vi "Laplace.vi"() -> ()   [LabVIEW 2021]
uses:
  <vilib>/Math Plots/3D Math Plots/3D Contour/3D Contour XCtrl/3D Contour.xctl
  <vilib>/Math Plots/3D Math Plots/3D Contour/3D Contour Datatype/Public/Plot Helper (Matrix).vi
  <vilib>/Math Plots/3D Math Plots/3D Contour/3D Contour Datatype/3D Contour Datatype.lvclass
panel:
  out "abs(x) 2":dbl[][](array[numeric])
  out "abs(x)":dbl
  out "Boolean":bool
  in  "Error":dbl
  out "3D Contour":refnum<class "3D Plot Datatype.lvclass">[](xcontrol)
  in  "dimension size":i32
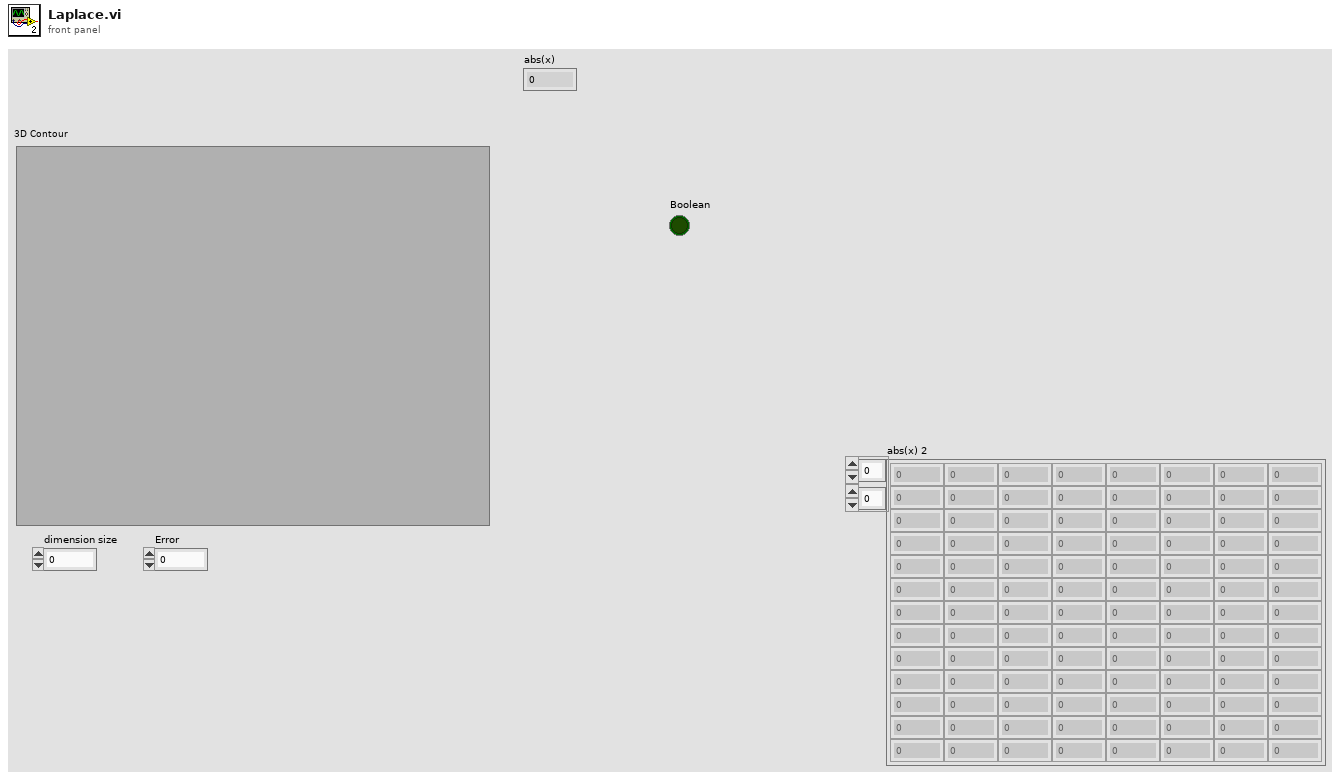
[diagram p1: front panel]
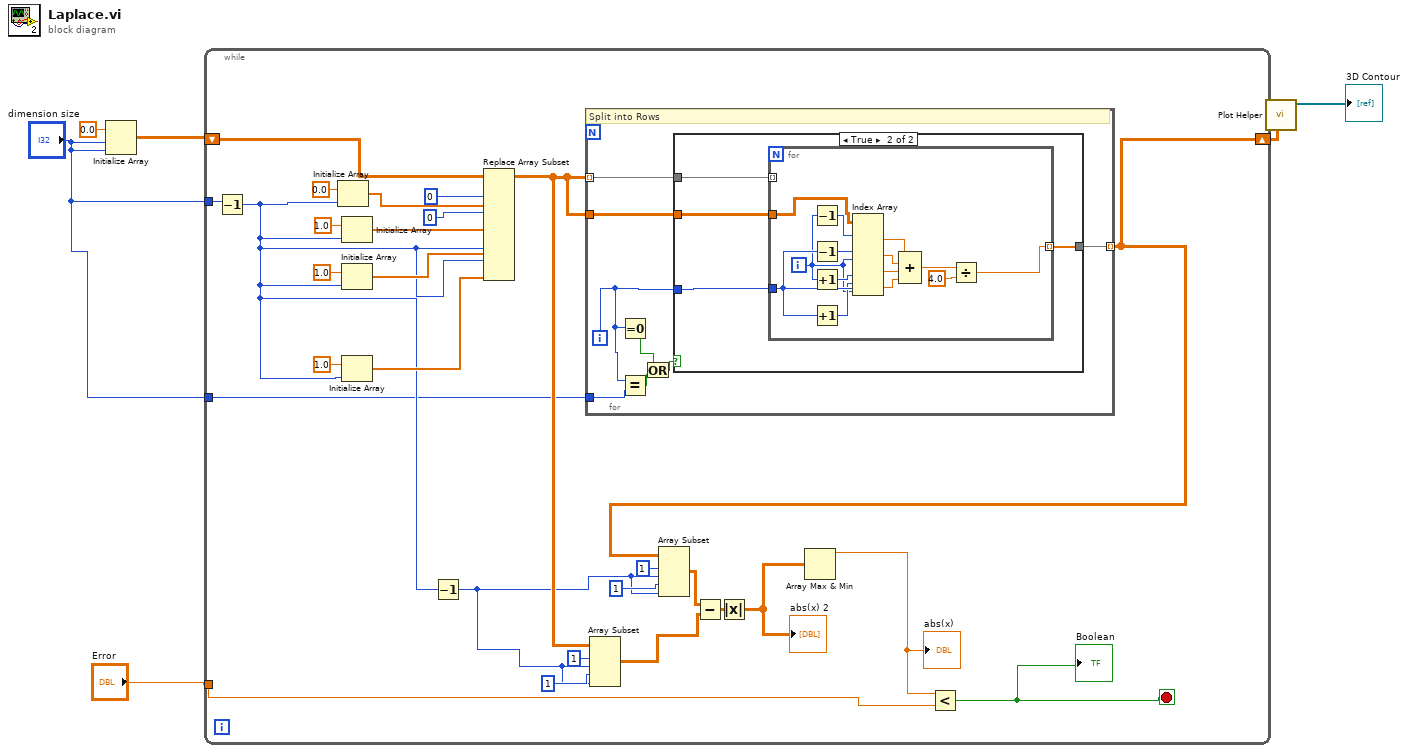
[diagram p0: block diagram]
diagram:
  n1 = Initialize Array(0.0 ("element"), "dimension size", "dimension size") -> (w5:dbl[][])
  n2 = while {
    tunnel: "dimension size" -> [w28]
    shift-right: [w12] -> w3
    shift-left: w5 -> [w29]
    tunnel: "Error" -> [w21]
    tunnel: "dimension size" -> [w7]
    stop <- w20 stop-if-true
    n3 = Decrement(x=w28) -> (x-1=w9:i32)
    n4 = Initialize Array(0.0 ("element"), w9) -> (w30:dbl[])
    n5 = Initialize Array(1.0 ("element"), w9) -> (w27:dbl[])
    n6 = Initialize Array(1.0 ("element"), w9) -> (w26:dbl[])
    n7 = Initialize Array(1.0 ("element"), w9) -> (w25:dbl[])
    n8 = Decrement(x=w9) -> (x-1=w8:i32)
    n9 = Replace Array Subset(array=w29, new element #1=w30, index (col) #1=0 ("index (row)"), new element #2=w27, index (row) #2=0 ("disabled index (col)"), new element #3=w26, index (col) #3=w9, new element #4=w25, index (row) #4=w9) -> (w10:dbl[][])  [unwired: 4 in]
    n10 = for {
      tunnel: w10 -> [w41] mode=indexing
      tunnel: [w42] -> w12 mode=indexing
      tunnel: w10 -> [w40]
      tunnel: w7 -> [w36]
      i -> [w35]
      # "Split into Rows"
      n11 = Equal To 0?(x=w35) -> (x = 0?=w39:bool)
      n12 = Equal?(x=w35, y=w36) -> (x = y?=w38:bool)
      n13 = Or(x=w39, y=w38) -> (x .or. y?=w37:bool)
      n14 = case shown="True" w37 {
        tunnel: [w43 w47] -> w42
        tunnel: w41 -> [w43 w46]
        tunnel: w40 -> [_ w45]
        tunnel: w35 -> [_ w44]
        frame False {
        }
        frame True {
          n15 = for {
            tunnel: w46 -> [_] mode=indexing
            tunnel: [w60] -> w47 mode=indexing
            tunnel: w44 -> [w52]
            tunnel: w45 -> [w57]
            i -> [w50]
            n16 = Decrement(x=w50) -> (x-1=w56:i32)
            n17 = Decrement(x=w52) -> (x-1=w55:i32)
            n18 = Increment(x=w50) -> (x+1=w53:i32)
            n19 = Increment(x=w52) -> (x+1=w51:i32)
            n20 = Index Array(array=w57, index (row) #1=w56, index (col) #1=w52, index (row) #2=w55, index (col) #2=w50, index (row) #3=w52, index (col) #3=w53, index (row) #4=w51, index (col) #4=w50) -> (element #1=w58:dbl, element #2=w54:dbl, element #3=w49:dbl, element #4=w48:dbl)
            n21 = Compound Arithmetic op=ADD(w58, w54, w49, w48) -> (w59:dbl)
            n22 = Divide(x=w59, y=4.0) -> (x/y=w60:dbl)
          }
        }
      }
    }
    n23 = Array Subset(array=w10, index (row)=1 ("index"), length (row)=w8, index (col)=1 ("index"), length (col)=w8) -> (w15:dbl[][])
    n24 = Array Subset(array=w12, index (row)=1 ("index"), length (row)=w8, index (col)=1 ("index"), length (col)=w8) -> (w11:dbl[][])
    n25 = Subtract(x=w11, y=w15) -> (x-y=w22:dbl[][])
    n26 = Absolute Value(x=w22) -> (abs(x)=w19:dbl[][])
    "abs(x) 2" <- w19
    n27 = Array Max & Min(array=w19) -> (max value=w18:dbl)  [unwired: 3 out]
    "abs(x)" <- w18
    n28 = Less?(x=w18, y=w21) -> (x < y?=w20:bool)
    "Boolean" <- w20
  }
  n29 = call-poly <vilib>:"Plot Helper.vi"("z matrix"=w3) -> ("3D Plot lvclass Array out"=→"3D Contour":refnum<class "3D Plot Datatype.lvclass">[])  [unwired: 5 in, 5 out]
